vi "RNN_Loss.vi"(1 "targets":i64[](array[numeric])=[0, 1], 4 "ps":dbl[][][](array[numeric])=[[[0.20328533], [0.10445738], [0.69225729]], [[0.24201603], [0.17203346], [0.58595051]]] format="%_8f") -> (15 "Loss (total)":dbl format="%_8f", 18 "Loss Array":dbl[](array[numeric]) format="%_8f")   [LabVIEW 2014]
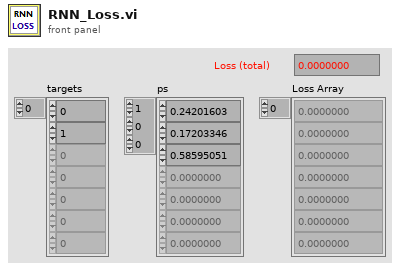
[diagram p1: front panel]
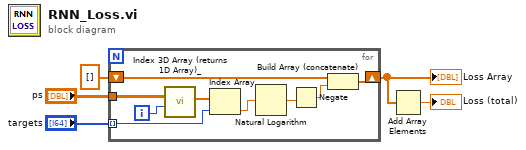
[diagram p0: block diagram]
diagram:
  n1 = for {
    tunnel: "ps" -> [w14]
    tunnel: "targets" -> [w11] mode=indexing
    shift-right: [w9] -> w1
    shift-left: dbl[] [] -> [w8]
    i -> [w13]
    n2 = call "Index 3D Array (returns 1D Array)_.vi"("index"=w13, "3D array"=w14) -> ("1D array"=w12:dbl[])  [unwired: 9 in]
    n3 = Index Array(array=w12, index=w11) -> (element=w7:dbl)
    n4 = Natural Logarithm(1:w7) -> (0:w10:dbl)
    n5 = Negate(x=w10) -> (-x=w6:dbl)
    n6 = Build Array (concatenate)(w8, w6) -> (w9:dbl[])
  }
  "Loss Array" <- w1
  n7 = Add Array Elements(numeric array=w1) -> (sum=→"Loss (total)":dbl)
